vi "Read ITC LPF Pressure.vi"(8 "error in (no error)":errorcluster, 11 "Instrument.Oxford1820 in":refnum<class "Instrument.OxfordVRM.lvclass">) -> (0 "error out":errorcluster, 2 "LPF Pressure (mbar)":dbl, 3 "Instrument.Oxford1820 out":refnum<class "Instrument.OxfordVRM.lvclass">)   [LabVIEW 2016]
uses:
  <instrlib>/Mercury iXX/Mercury iXX.lvlib
  <instrlib>/Mercury iXX/Public/Libraries/Pressure/Configuration/Read/Pressure Device (Read).vi
  <instrlib>/Mercury iXX/Public/Libraries/Pressure.lvlib
  <instrlib>/Mercury iXX/Public/Libraries/Pressure/Open/Open Pressure Device.vi
  Instrument.OxfordVRM.lvclass
  C:/Program Files (x86)/National Instruments/LabVIEW 2016/user.lib/LevyLab/Levylab Instruments/Instrument Types/Cryostat/Instrument.Cryostat.lvclass
  C:/Program Files (x86)/National Instruments/LabVIEW 2016/user.lib/LevyLab/Levylab Instruments/SMOs/Instrument/Instrument.lvclass
  C:/Program Files (x86)/National Instruments/LabVIEW 2016/vi.lib/JKI/JKI SMO/SMO/SMO.lvclass
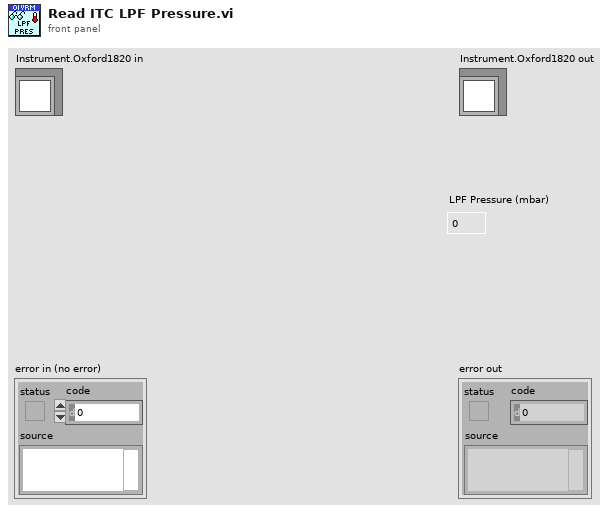
[diagram p1: front panel]
types:
  T1 = typedef "Mercury iXX.lvlib/Mercury Reference.ctl" = cluster{"Comms":refnum<visa-resource-name>, "Device ID":string[], "Comms Layer":T2, "Command":string, "Query reference":T3}
  T2 = typedef "Mercury iXX.lvlib/Comms Transport Layer.ctl" = enum16{"Ethernet TCP/IP", "USB", "ISOBus - RS-232", "GPIB"}
  T3 = typedef "Mercury iXX.lvlib/Query Dynamic Reference.ctl" = refnum<vi>
  T4 = typedef "Mercury iXX.lvlib/Pressure.lvlib/Pressure Device (Read).ctl" = cluster{"Manufacturing":T5, "Temperature Sensor Type":T6, "Calibration":T7, "Control Loop":T9, "Pressure Signals":T10, "Nickname":string, "Status":string}
  T5 = typedef "Mercury iXX.lvlib/Manufacturing Data.ctl" = cluster{"Hardware Version":string, "Firmware Version":string, "Serial Number":string}
  T6 = typedef "Mercury iXX.lvlib/Pressure.lvlib/Pressure Sensor Type.ctl" = string
  T7 = typedef "Mercury iXX.lvlib/Pressure.lvlib/Calibration Cluster.ctl" = cluster{"Filename":string, "Interpolation":T8, "Scaling Factor":string, "Offset Factor":string, "High Limit":string, "Low Limit":string, "Last Calibration":string}
  T8 = typedef "Mercury iXX.lvlib/Pressure.lvlib/Calibration Interpolation.ctl" = string
  T9 = typedef "Mercury iXX.lvlib/Pressure.lvlib/Loop Cluster.ctl" = cluster{"Heater":string, "Auxiliary":string, "Heater Auto":string, "Percentage Heat":string, "Pressure Set Point":string, "PID Auto (from file)":string, "P Value":string, "I Value":string, "D Value":string, "Auto PID Table Filename":string, "Flow Auto":string, "Target Heater Table":string, "Sweep mode":string, "Sweep Table Filename":string, "Percentage Flow":string}
  T10 = typedef "Mercury iXX.lvlib/Pressure.lvlib/Pressure Signals Cluster.ctl" = cluster{"Voltage":string, "Current":string, "Power":string, "Pressure":string}
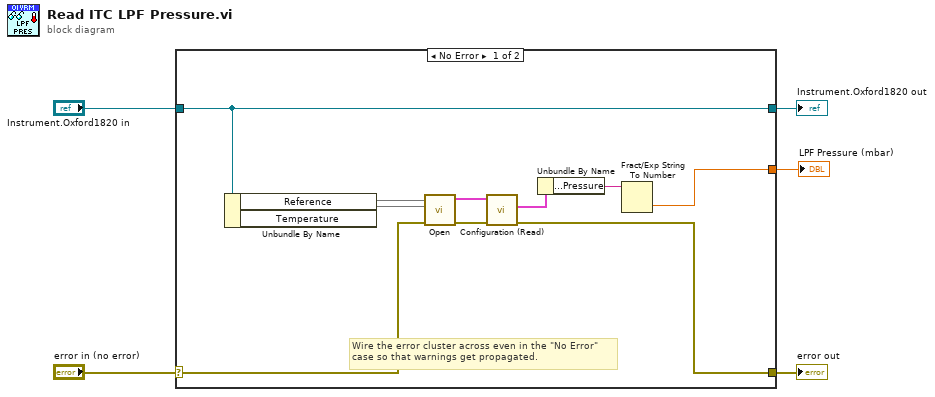
[diagram p0: block diagram]
diagram:
  n1 = case shown="No Error" "error in (no error)" {
    selector: "error in (no error)" -> [w9 w17]
    tunnel: [w6 w17] -> w4
    tunnel: [w15 w16] -> w2
    tunnel: "Instrument.Oxford1820 in" -> [w15 w16]
    tunnel: [w7 _] -> w1
    frame No Error {
      # "Wire the error cluster across even in the \"No Error\"\ncase so that warnings get propagated."
      n2 = Unbundle By Name(w15) -> ("Reference"=w11, "Temperature"=w10)
      n3 = call-poly <instrlib>:"Open.vi"("error in (no error)"=w9, "Device Identifier"=w10, "Mercury Reference In"=w11) -> ("error out"=w14:errorcluster, "Mercury Reference Out"=w13:T1)  [unwired: 7 out]
      n4 = call-poly <instrlib>:"Configuration (Read).vi"("error in"=w14, "Mercury Reference In"=w13) -> ("error out"=w6:errorcluster, "Device Details"=w8:T4)  [unwired: 1 in, 7 out]
      n5 = Unbundle By Name(w8) -> ("Pressure Signals.Pressure"=w12:string)
      n6 = Fract/Exp String To Number(string=w12) -> (number=w7:dbl)  [unwired: 3 in, 1 out]
    }
    frame Error {
    }
  }
  "error out" <- w4
  "Instrument.Oxford1820 out" <- w2
  "LPF Pressure (mbar)" <- w1
